vi "Write Obs.vi"(8 "error in (no error)":errorcluster, 10 "Obs":u16, 11 "Obs Based Step in":refnum<class "Obs Based Step.lvclass">) -> (0 "error out":errorcluster, 3 "Obs Based Step out":refnum<class "Obs Based Step.lvclass">)   [LabVIEW 2015, in "Obs Based Step.lvclass"]
uses:
  Obs Based Step.lvclass
  Obs Based Step.lvclass/Obs Based Step.ctl
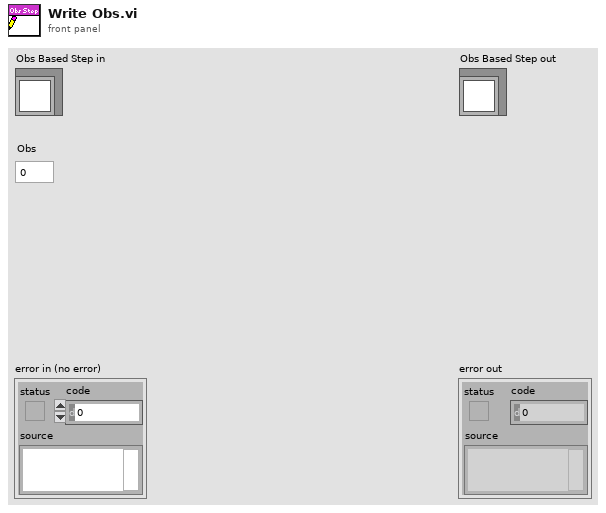
[diagram p1: front panel]
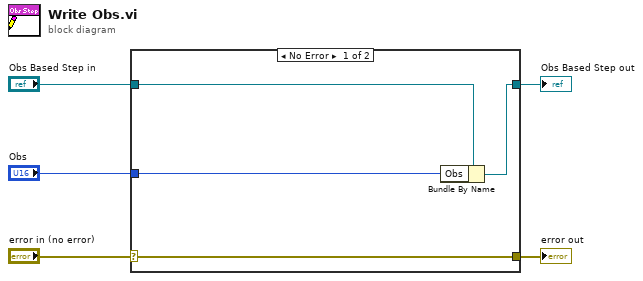
[diagram p0: block diagram]
diagram:
  n1 = case shown="No Error" "error in (no error)" {
    selector: "error in (no error)" -> [w9 w10]
    tunnel: [w9 w10] -> w4
    tunnel: [w7 w11] -> w2
    tunnel: "Obs Based Step in" -> [w8 w11]
    tunnel: "Obs" -> [w6 _]
    frame No Error {
      n2 = Bundle By Name(cluster=w8, "Obs"=w6) -> (w7:refnum<class "Obs Based Step.lvclass">)
    }
    frame Error {
    }
  }
  "error out" <- w4
  "Obs Based Step out" <- w2
